vi "Read Stdout.vi"(8 "error in":errorcluster, 10 "byte count":i32, 11 "pipe in":T1) -> (0 "error out":errorcluster, 1 "return count":i32, 2 "read buffer":string, 3 "pipe out":T1, 4 "exited":bool, 5 "bytes remaining":i32)   [LabVIEW 2013, in "LV Process library.lvlib"]
doc: "Calls lv_proc.dll to read stdout of a process and returns read buffer. Also returns count of remaining bytes in the pipe and process status."
uses:
  LV Process library.lvlib
  Pipe Handle.ctl
panel:
  in  "exit mem":i32
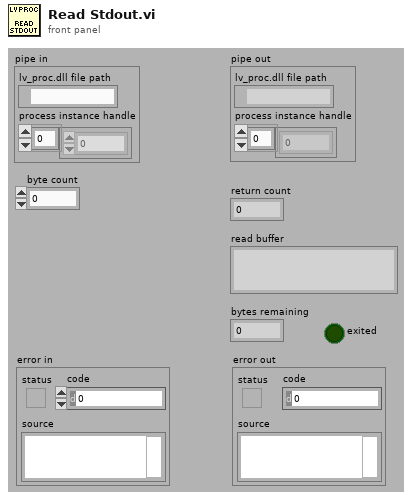
[diagram p1: front panel]
types:
  T1 = typedef "LV Process library.lvlib/Pipe Handle.ctl" = cluster{"lv_proc.dll file path":path, "process instance handle":u32[]}
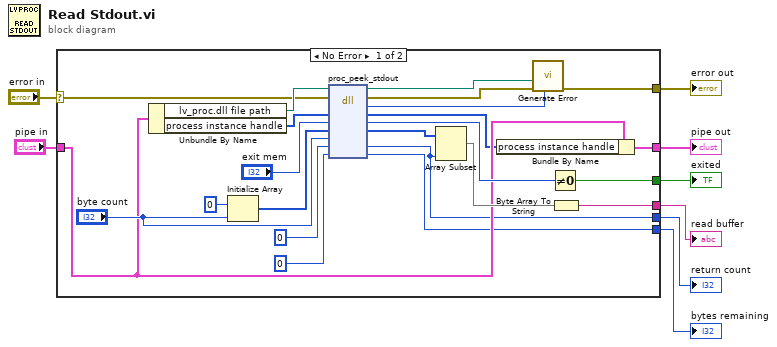
[diagram p0: block diagram]
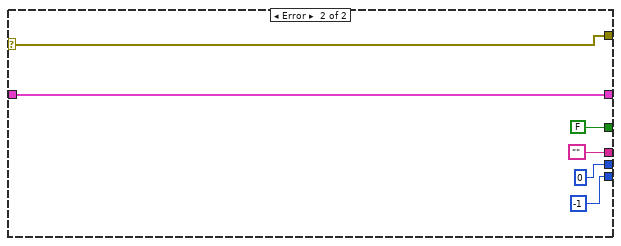
[diagram p2: hidden frame]
diagram:
  n1 = case shown="No Error" "error in" {
    selector: "error in" -> [w13 w37]
    tunnel: [w21 w36] -> w8
    tunnel: "pipe in" -> [w20 w36]
    tunnel: [w14 w37] -> w6
    tunnel: [w12 ""] -> w4
    tunnel: [w11 FALSE] -> w3
    tunnel: [w10 0 ("read")] -> w2
    tunnel: [w9 -1 ("toread")] -> w1
    frame No Error {
      n2 = Unbundle By Name(w20) -> ("lv_proc.dll file path"=w22:path, "process instance handle"=w17:u32[])
      n3 = Initialize Array(u8 0 ("element"), "byte count") -> (w28:u8[])
      n4 = dll-call lib="lv_proc.dll" fn="proc_peek_stdout"(path in=w22, error in=w13, "proc"=w17, "exit"="exit mem", "buffer"=w28, "size"="byte count", "read"=0 ("read mem"), "toread"=0 ("toread mem")) -> (path out=w16:path, error out=w15:errorcluster, "error"=w18:i32, "proc"=w19:u32[], "exit"=w25:i32, "buffer"=w24:u8[], "read"=w10:i32, "toread"=w9:i32)  [unwired: 2 in]
      n5 = Array Subset(array=w24, length=w10) -> (w23:u8[])  [unwired: 1 in]
      n6 = Bundle By Name(cluster=w20, "process instance handle"=w19) -> (w21:T1)
      n7 = call "Generate Error.vi"("error code in"=w18, "error in"=w15, "lv_proc.dll path in"=w16) -> ("error out"=w14:errorcluster)  [unwired: 6 in, 1 out]
      n8 = Not Equal To 0?(x=w25) -> (x != 0?=w11:bool)
      n9 = Byte Array To String(unsigned byte array=w23) -> (string=w12:string)
    }
    frame Error {
    }
  }
  "error out" <- w6
  "pipe out" <- w8
  "read buffer" <- w4
  "exited" <- w3
  "return count" <- w2
  "bytes remaining" <- w1
